vi "CLD 12 Sequencer State Machine.vi"() -> ()   [LabVIEW 2018]
doc: "CLD 12 exercise"
uses:
  CLD 12 Sequencer Enum.ctl
  CLD 12 Data Cluster.ctl
  CLD12 Timer Enum.ctl
panel:
  out "Current Time Target":dbl
  in  "Stop Button":bool
  out "Time Elapsed":dbl
  out "Switch 3":bool
  out "Switch 2":bool
  out "Switch 1":bool
  in  "Start":bool
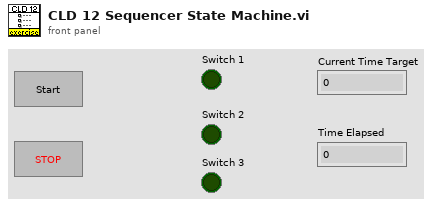
[diagram p1: front panel]
types:
  T1 = typedef "CLD 12 Data Cluster.ctl" = cluster{"Command":T2, "Time Value":dbl, "Boolean 1":bool, "Boolean 2":bool, "Boolean 3":bool}
  T2 = typedef "CLD 12 Sequencer Enum.ctl" = enum16{"Initialize", "SetTime", "RunState1", "Runstate2", "Idle", "Start"}
  T3 = typedef "CLD12 Timer Enum.ctl" = enum16{"Start Timer", "Read Time", "Pause", "UnPause", "Reset Timer"}
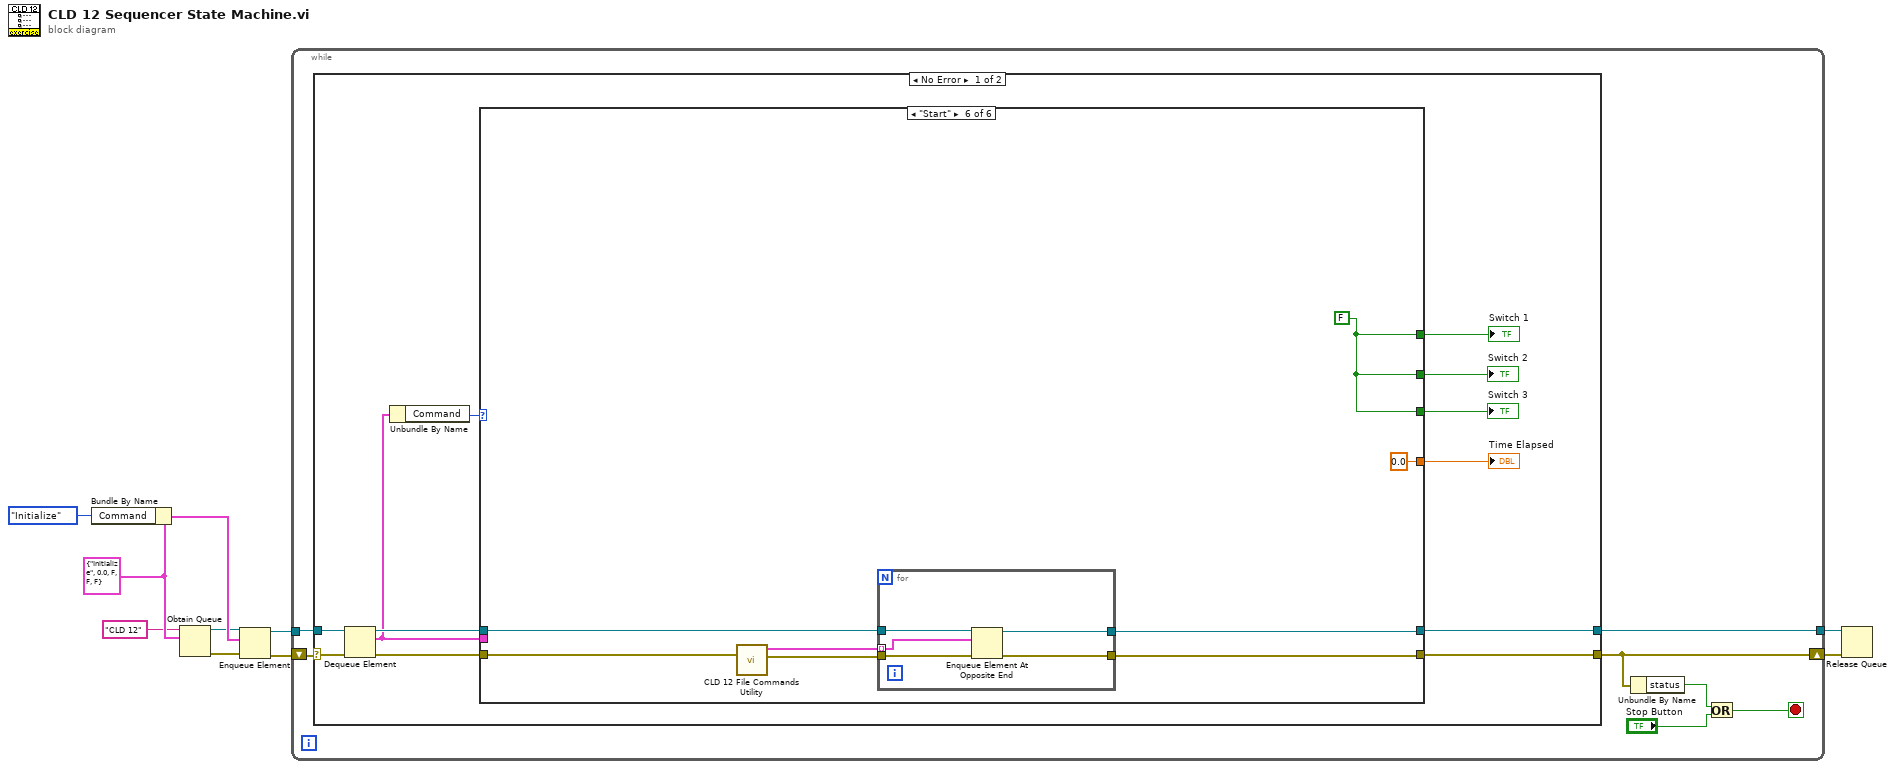
[diagram p0: block diagram]
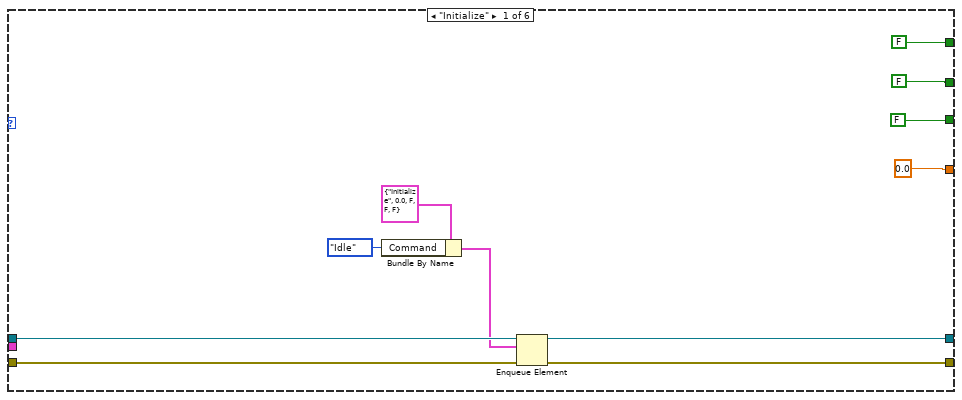
[diagram p2: hidden frame]
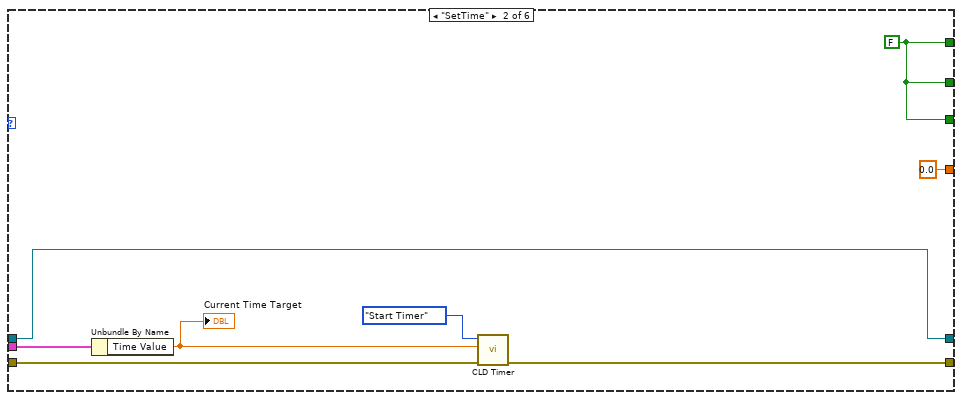
[diagram p3: hidden frame]
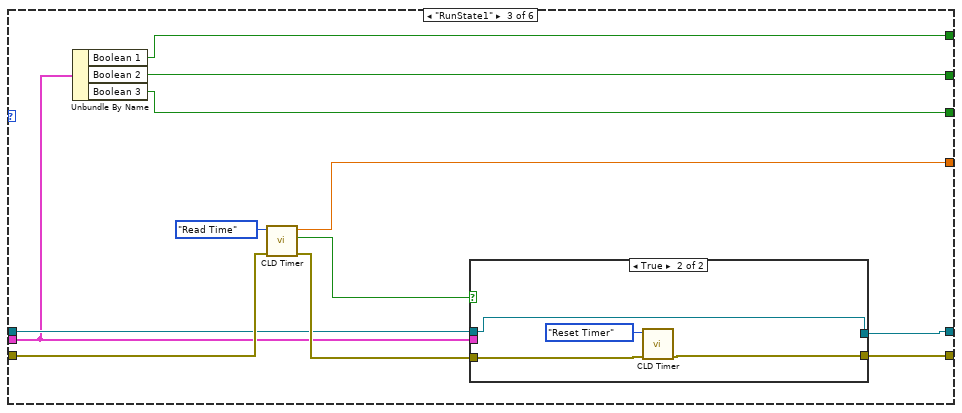
[diagram p4: hidden frame]
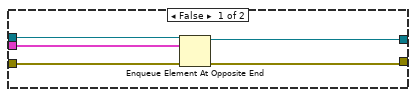
[diagram p5: hidden frame]
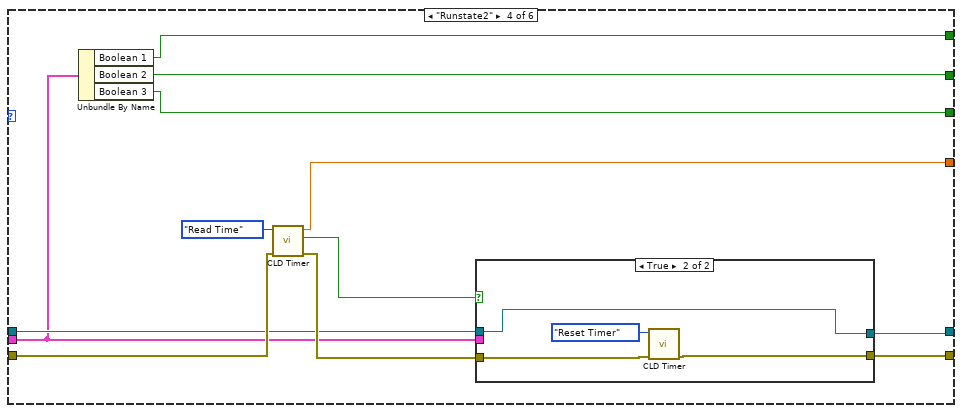
[diagram p6: hidden frame]
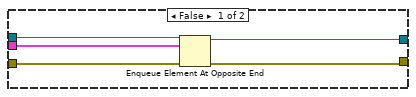
[diagram p7: hidden frame]
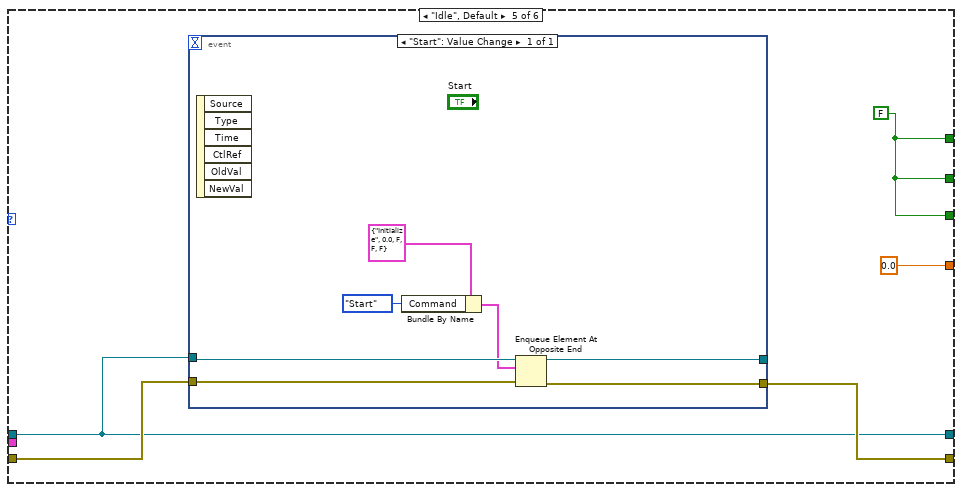
[diagram p8: hidden frame]
diagram:
  w10 = T1 {"Command"=enum."Initialize", "Time Value"=0.0, "Boolean 1"=FALSE, "Boolean 2"=FALSE, "Boolean 3"=FALSE} ("CLD 12 Data Cluster")
  n1 = Bundle By Name(cluster=w10, "Command"=CLD_12_Sequencer_Enum."Initialize" ("CLD 12 Sequencer Control")) -> (w8:T1)
  n2 = Obtain Queue(name (unnamed)="CLD 12", element data type=w10) -> (queue out=w7:refnum<queue>, error out=w6:errorcluster)  [unwired: 3 in, 1 out]
  n3 = Enqueue Element(queue=w7, element=w8, error in (no error)=w6) -> (queue out=w3:refnum<queue>, error out=w4:errorcluster)  [unwired: 1 in, 1 out]
  n4 = while {
    tunnel: w3 -> [w16]
    shift-right: [w14] -> w2
    shift-left: w4 -> [w17]
    tunnel: [w15] -> w1
    stop <- w11 stop-if-true
    n5 = case shown="No Error" w17 {
      selector: w17 -> [w29 w116]
      tunnel: w16 -> [w28 w117]
      tunnel: [w21 w116] -> w14
      tunnel: [w18 w117] -> w15
      frame No Error {
        n6 = Dequeue Element(queue=w28, error in (no error)=w29) -> (queue out=w20:refnum<queue>, element=w19:T1, error out=w22:errorcluster)  [unwired: 1 in, 1 out]
        n7 = Unbundle By Name(w19) -> ("Command"=w27:T2)
        n8 = case shown="\"Start\"" w27 {
          tunnel: [FALSE w42 w55 w73 w93 w104] -> w26
          tunnel: [FALSE w42 w56 w74 w93 w104] -> w25
          tunnel: [FALSE w42 w54 w72 w93 w104] -> w24
          tunnel: [0.0 0.0 ("Elapsed Time") w53 w75 0.0 0.0] -> w23
          tunnel: w22 -> [w36 w48 w60 w78 w95 w110]
          tunnel: [w35 w47 w50 w71 w94 w109] -> w21
          tunnel: w20 -> [w34 w45 w52 w77 w91 w107]
          tunnel: w19 -> [_ w46 w51 w76 _ _]
          tunnel: [w30 w45 w49 w70 w91 w105] -> w18
          frame "Initialize" {
            n9 = Bundle By Name(cluster=T1 {"Command"=enum."Initialize", "Time Value"=0.0, "Boolean 1"=FALSE, "Boolean 2"=FALSE, "Boolean 3"=FALSE} ("element"), "Command"=CLD_12_Sequencer_Enum."Idle") -> (w31:T1)
            n10 = Enqueue Element(queue=w34, element=w31, error in (no error)=w36) -> (queue out=w30:refnum<queue>, error out=w35:errorcluster)  [unwired: 1 in, 1 out]
          }
          frame "SetTime" {
            w42 = FALSE
            n11 = Unbundle By Name(w46) -> ("Time Value"=w44:dbl)
            "Current Time Target" <- w44
            n12 = call "CLD Timer.vi"("error in"=w48, "Time Target (s)"=w44, "CLD 12 Timer Enum"=CLD12_Timer_Enum."Start Timer") -> ("error out"=w47:errorcluster)  [unwired: 6 in, 2 out]
          }
          frame "RunState1" {
            n13 = Unbundle By Name(w51) -> ("Boolean 1"=w55:bool, "Boolean 2"=w56:bool, "Boolean 3"=w54:bool)
            n14 = call "CLD Timer.vi"("error in"=w60, "CLD 12 Timer Enum"=CLD12_Timer_Enum."Read Time") -> ("error out"=w59:errorcluster, "Has Time Elapsed?"=w58:bool, "Elapsed Time"=w53:dbl)  [unwired: 7 in]
            n15 = case shown="True" w58 {
              tunnel: w59 -> [w65 w69]
              tunnel: w52 -> [w62 w67]
              tunnel: w51 -> [w63 _]
              tunnel: [w64 w68] -> w50
              tunnel: [w61 w67] -> w49
              frame False {
                n16 = Enqueue Element At Opposite End(queue=w62, element=w63, error in (no error)=w65) -> (queue out=w61:refnum<queue>, error out=w64:errorcluster)  [unwired: 1 in, 1 out]
              }
              frame True {
                n17 = call "CLD Timer.vi"("error in"=w69, "CLD 12 Timer Enum"=CLD12_Timer_Enum."Reset Timer") -> ("error out"=w68:errorcluster)  [unwired: 7 in, 2 out]
              }
            }
          }
          frame "Runstate2" {
            n18 = Unbundle By Name(w76) -> ("Boolean 1"=w73:bool, "Boolean 2"=w74:bool, "Boolean 3"=w72:bool)
            n19 = call "CLD Timer.vi"("error in"=w78, "CLD 12 Timer Enum"=CLD12_Timer_Enum."Read Time") -> ("error out"=w81:errorcluster, "Has Time Elapsed?"=w80:bool, "Elapsed Time"=w75:dbl)  [unwired: 7 in]
            n20 = case shown="True" w80 {
              tunnel: w81 -> [w86 w90]
              tunnel: [w85 w89] -> w71
              tunnel: [w84 w87] -> w70
              tunnel: w76 -> [w82 _]
              tunnel: w77 -> [w83 w87]
              frame False {
                n21 = Enqueue Element At Opposite End(queue=w83, element=w82, error in (no error)=w86) -> (queue out=w84:refnum<queue>, error out=w85:errorcluster)  [unwired: 1 in, 1 out]
              }
              frame True {
                n22 = call "CLD Timer.vi"("error in"=w90, "CLD 12 Timer Enum"=CLD12_Timer_Enum."Reset Timer") -> ("error out"=w89:errorcluster)  [unwired: 7 in, 2 out]
              }
            }
          }
          frame "Idle", Default {
            w93 = FALSE
            n23 = event shown="[0] \"Start\": Value Change" {
              selector: _ -> [_]
              dyn-events: _ -> [_]
              timeout: _ -> [_]
              tunnel: w95 -> [w102]
              tunnel: w91 -> [w100]
              tunnel: [w101] -> w94
              tunnel: [w96] -> _
              event "Start": Value Change {
                n24 = event-data() -> ()  [unwired: 1 in, 6 out]
                n25 = Bundle By Name(cluster=T1 {"Command"=enum."Initialize", "Time Value"=0.0, "Boolean 1"=FALSE, "Boolean 2"=FALSE, "Boolean 3"=FALSE} ("CLD 12 Data Cluster"), "Command"=CLD_12_Sequencer_Enum."Start") -> (w97:T1)
                n26 = Enqueue Element At Opposite End(queue=w100, element=w97, error in (no error)=w102) -> (queue out=w96:refnum<queue>, error out=w101:errorcluster)  [unwired: 1 in, 1 out]
              }
            }
          }
          frame "Start" {
            w104 = FALSE
            n27 = call "CLD 12 File Commands Utility.vi"("Error In"=w110) -> ("Error Out"=w106:errorcluster, "Commands Out Array"=w108:T1[])  [unwired: 6 in]
            n28 = for {
              tunnel: w108 -> [w113] mode=indexing
              tunnel: w106 -> [w115]
              tunnel: [w114] -> w109
              tunnel: w107 -> [w112]
              tunnel: [w111] -> w105
              n29 = Enqueue Element At Opposite End(queue=w112, element=w113, error in (no error)=w115) -> (queue out=w111:refnum<queue>, error out=w114:errorcluster)  [unwired: 1 in, 1 out]
            }
          }
        }
        "Switch 3" <- w24
        "Switch 2" <- w25
        "Switch 1" <- w26
        "Time Elapsed" <- w23
      }
      frame Error {
      }
    }
    n30 = Unbundle By Name(w14) -> ("status"=w13:bool)
    n31 = Or(x=w13, y="Stop Button") -> (x .or. y?=w11:bool)
  }
  n32 = Release Queue(queue=w1, error in (no error)=w2) -> ()  [unwired: 1 in, 3 out]
